vi "StopTask.vi"(8 "error in (no error)":errorcluster, 11 "NI_DAQmx(Angular) in":refnum<class "NI_DAQmx(Angular).lvclass">) -> (0 "error out":errorcluster, 3 "NI_DAQmx(Angular) out":refnum<class "NI_DAQmx(Angular).lvclass">)   [LabVIEW 2025, in "NI_DAQmx(Angular).lvclass"]
uses:
  NI_DAQmx(Angular).lvclass
  NI_DAQmx(Angular).lvclass/NI_DAQmx(Angular).ctl
  DAQ_Abstr/Task_Type/Angular_Task/Angular_Task/Angular_Task.lvclass
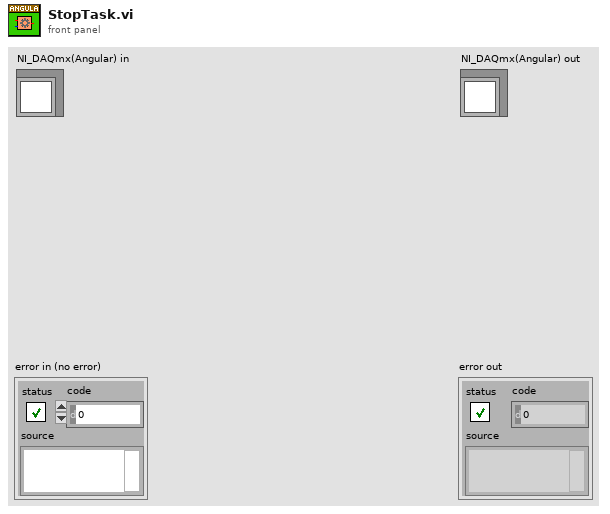
[diagram p1: front panel]
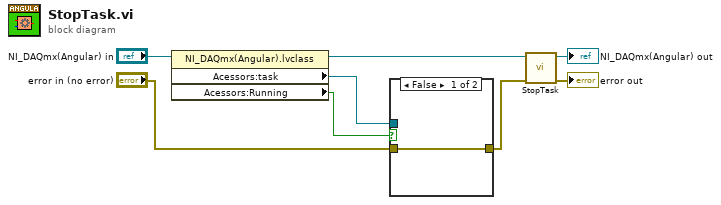
[diagram p0: block diagram]
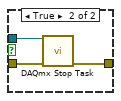
[diagram p2: hidden frame]
diagram:
  n1 = property class="NI_DAQmx(Angular).lvclass"(reference="NI_DAQmx(Angular) in") -> (reference out=w3:refnum<class "NI_DAQmx(Angular).lvclass">, "Acessors:task"=w6:refnum<k21>, "Acessors:Running"=w5:bool)  [unwired: 1 in, 1 out]
  n2 = case shown="False" w5 {
    tunnel: w6 -> [_ w12]
    tunnel: [w9 w11] -> w1
    tunnel: "error in (no error)" -> [w9 w10]
    frame False {
    }
    frame True {
      n3 = call <vilib>:"DAQmx Stop Task.vi"("task/channels in"=w12, "error in"=w10) -> ("error out"=w11:errorcluster)  [unwired: 12 in, 1 out]
    }
  }
  n4 = call-parent "StopTask.vi"("error in (no error)"=w1, "Task_Abstr in"=w3) -> ("error out"=→"error out":errorcluster, "Task_Abstr out"=→"NI_DAQmx(Angular) out":refnum<class "NI_DAQmx(Angular).lvclass">)  [unwired: 8 in]
